vi "Curva Linear Calibracao.vi"(1 "input type":u16(ring)=1 items=["tensao", "corrente"], 2 "MIN":i32, 3 "MAX":i32, 4 "input":dbl) -> (0 "output":dbl)   [LabVIEW 2019]
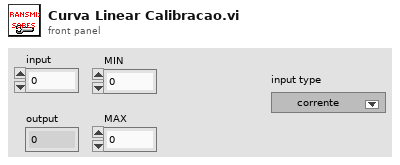
[diagram p1: front panel]
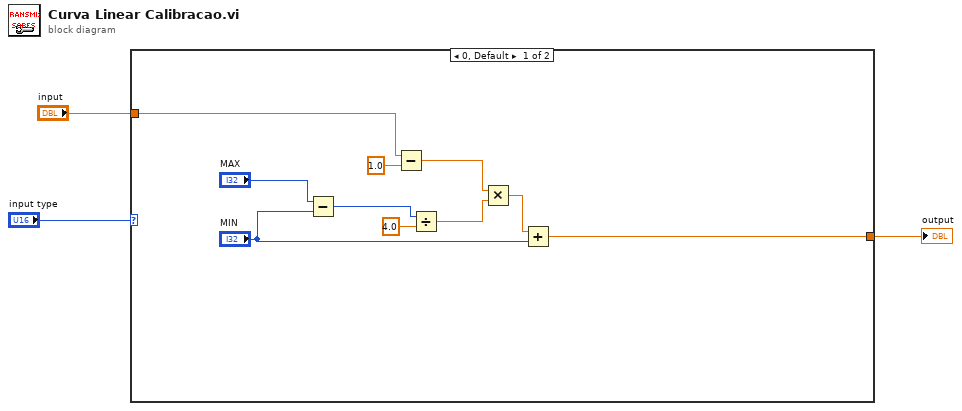
[diagram p0: block diagram]
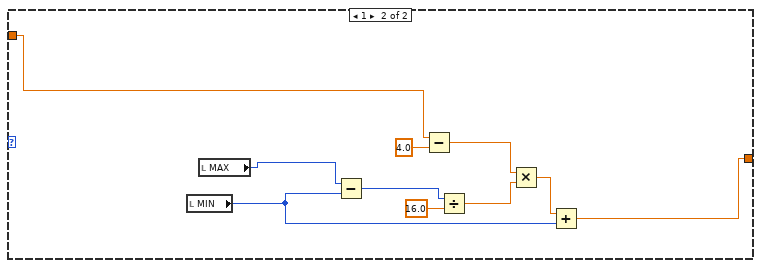
[diagram p2: hidden frame]
diagram:
  n1 = case shown="0, Default" "input type" {
    tunnel: [w5 w17] -> w3
    tunnel: "input" -> [w4 w14]
    frame 0, Default {
      n2 = Subtract(x="MAX", y="MIN") -> (x-y=w12:i32)
      n3 = Subtract(x=w4, y=1.0) -> (x-y=w9:dbl)
      n4 = Divide(x=w12, y=4.0) -> (x/y=w8:dbl)
      n5 = Multiply(x=w9, y=w8) -> (x*y=w7:dbl)
      n6 = Add(x=w7, y="MIN") -> (x+y=w5:dbl)
    }
    frame 1 {
      n7 = local read "MIN"() -> (w16:i32)
      n8 = local read "MAX"() -> (w15:i32)
      n9 = Subtract(x=w15, y=w16) -> (x-y=w23:i32)
      n10 = Subtract(x=w14, y=4.0) -> (x-y=w20:dbl)
      n11 = Divide(x=w23, y=16.0) -> (x/y=w19:dbl)
      n12 = Multiply(x=w20, y=w19) -> (x*y=w18:dbl)
      n13 = Add(x=w18, y=w16) -> (x+y=w17:dbl)
    }
  }
  "output" <- w3
